vi "logoff tcp.vi"(8 "error in (no error)":errorcluster, 11 "Connection ID":refnum<k5>) -> (0 "error out":errorcluster, 3 "Connection ID out":refnum<k5>)   [LabVIEW 2019]
doc: "Logs off of the data server and returns any error codes.\n\nInputs\n\nConnection ID - TCP connection that is to be terminated.\n\nOutputs\n\nError out - Error codes generated during logoff.\n\nCreated by Monroe Weber-Shirk\nCornell University\nmw24@cornell.edu\nJanuary 2000"
uses:
  DataServer/command cluster.ctl
  DataServer/command.ctl
panel:
  in  "command interface":T1={"command"=enum."Logoff", "start time (ms)"=0, "Channel Indices"=[], "Scans per Sample"=1} {"Scans per Sample" min=1}
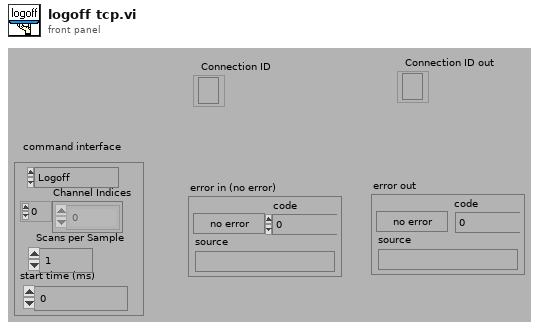
[diagram p1: front panel]
types:
  T1 = typedef "command cluster.ctl" = cluster{"command":T2, "start time (ms)":u32, "Channel Indices":i32[], "Scans per Sample":i32}
  T2 = typedef "command.ctl" = enum16{"Idle", "Send Data", "Send 1 Scan", "Logoff"}
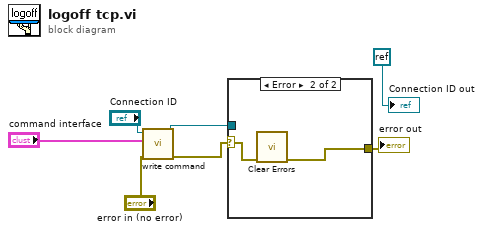
[diagram p0: block diagram]
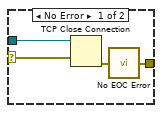
[diagram p2: hidden frame]
diagram:
  n1 = call "write command.vi"("error in (no error)"="error in (no error)", "command interface"="command interface", "refnum in"="Connection ID") -> ("error out"=w2:errorcluster, "refnum out"=w7:refnum<k5>)  [unwired: 7 in]
  n2 = case shown="Error" w2 {
    selector: w2 -> [w8 w13]
    tunnel: w7 -> [w11 _]
    tunnel: [w9 w12] -> w3
    frame No Error {
      n3 = TCP Close Connection(connection ID=w11, error in (no error)=w8) -> (error out=w10:errorcluster)  [unwired: 1 in, 1 out]
      n4 = call "No EOC Error.vi"("error in"=w10) -> ("error out"=w9:errorcluster)  [unwired: 4 in]
    }
    frame Error {
      n5 = call <vilib>:"Clear Errors.vi"("error in (no error)"=w13) -> ("error out"=w12:errorcluster)  [unwired: 5 in, 1 out]
    }
  }
  "error out" <- w3
  "Connection ID out" <- refnum<k0> refnum
